vi "IR sensor Subvi.vi"(8 "Numeric":dbl) -> (9 "Connected?":bool)   [LabVIEW 2019]
panel:
  out "Voltage":dbl
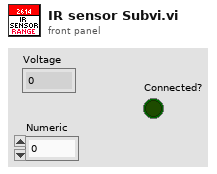
[diagram p1: front panel]
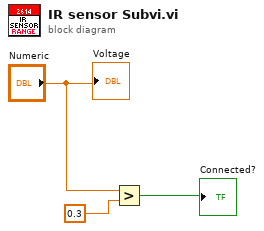
[diagram p0: block diagram]
diagram:
  n1 = Greater?(x="Numeric", y=0.3) -> (0:→"Connected?":bool)
  "Voltage" <- "Numeric"
